vi "Get Actuator Position.vi"() -> (0 "Actuator Position":dbl)   [LabVIEW 2011]
uses:
  Globals/Actuator Home Position.vi
  Globals/Potentiometers.vi
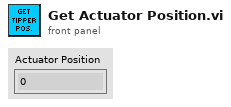
[diagram p1: front panel]
types:
  T1 = typedef "WPI_AnalogChannelDevRef.ctl" = cluster{"DevStatus":errorcluster, "Analog Module":T2, "Analog Channel":T3}
  T2 = typedef "FPGA_TypedefAnalogModule.ctl" = enum16{"Analog Module 1", "Analog Module 2"}
  T3 = typedef "FPGA_AIChannel.ctl" = enum8{"AI 1", "AI 2", "AI 3", "AI 4", "AI 5", "AI 6", "AI 7", "AI 8", "Invalid"}
  T4 = cluster{"Front Left":T1, "Front Right":T1, "Rear Left":T1, "Rear Right":T1, "Actuator":T1}
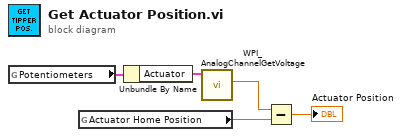
[diagram p0: block diagram]
diagram:
  n1 = global read "Potentiometers.vi" "Potentiometers"() -> (w3:T4)
  n2 = global read "Actuator Home Position.vi" "Actuator Home Position"() -> (w5:dbl)
  n3 = Unbundle By Name(w3) -> ("Actuator"=w2:T1)
  n4 = call <vilib>:"WPI_AnalogChannelGetVoltage.vi"("AIDeviceRef"=w2) -> ("Voltage"=w1:dbl)  [unwired: 8 in, 2 out]
  n5 = Subtract(x=w1, y=w5) -> (x-y=→"Actuator Position":dbl)
